vi "Construct.vi"(8 "error in (no error)":errorcluster, 9 "Topic":string, 10 "Subscription ID":u64, 11 "SubscriptionDetails JSON in":refnum<class "SubscriptionDetails JSON.lvclass">) -> (0 "error out":errorcluster, 3 "SubscriptionDetails JSON out":refnum<class "SubscriptionDetails JSON.lvclass">)   [LabVIEW 2020, in "wamplv.lvlib" / "SubscriptionDetails JSON.lvclass"]
uses:
  SubscriptionDetails JSON.lvclass
  SubscriptionDetails JSON.lvclass/SubscriptionDetails JSON.ctl
  SubscriptionDetailsParent/SubscriptionDetailsParent.lvclass
  WAMP Client/Private/TypeDef/EVENT payload (JSON).ctl
  wamplv.lvlib
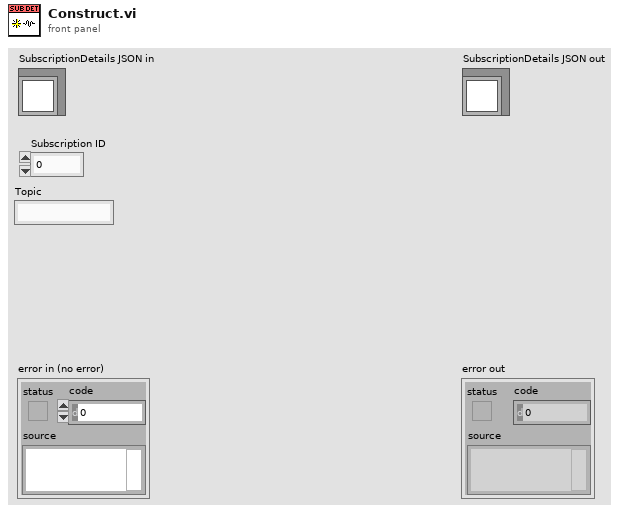
[diagram p1: front panel]
types:
  T1 = typedef "wamplv.lvlib/EVENT payload (JSON).ctl" = cluster{"Publication ID":u64, "Topic":string, "Arguments Payload":string, "ArgumentKw Payload":string, "Details":string}
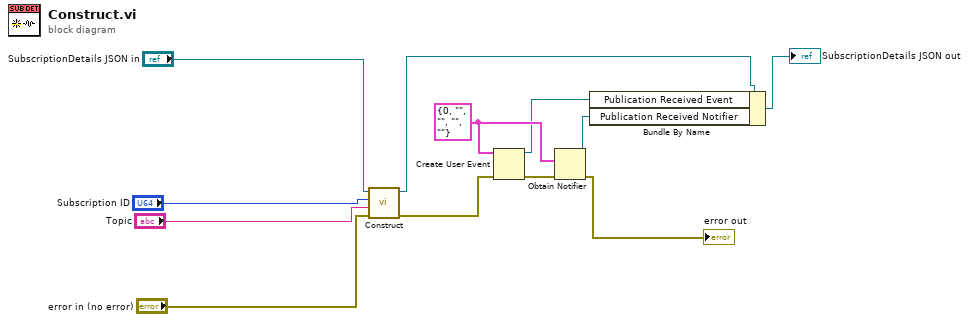
[diagram p0: block diagram]
diagram:
  w8 = T1 {"Publication ID"=0, "Topic"="", "Arguments Payload"="", "ArgumentKw Payload"="", "Details"=""} ("Cluster")
  n1 = call-parent "Construct.vi"("error in (no error)"="error in (no error)", "Topic"="Topic", "Subscription ID"="Subscription ID", "SubscriptionDetailsParent in"="SubscriptionDetails JSON in") -> ("error out"=w2:errorcluster, "SubscriptionDetailsParent out"=w4:refnum<class "SubscriptionDetails JSON.lvclass">)  [unwired: 6 in]
  n2 = Create User Event(user event datatype=w8, error in=w2) -> (user event=w6:refnum<user-event>, error out=w7:errorcluster)
  n3 = Obtain Notifier(notification data type=w8, error in (no error)=w7) -> (notifier out=w5:refnum<notifier>, error out=→"error out":errorcluster)  [unwired: 2 in, 1 out]
  n4 = Bundle By Name(cluster=w4, "Publication Received Event"=w6, "Publication Received Notifier"=w5) -> (→"SubscriptionDetails JSON out":refnum<class "SubscriptionDetails JSON.lvclass">)
